vi "ScoutingMain.vi"() -> ()   [LabVIEW 2017]
uses:
  <vilib>/Utility/NIReport.llb/Append Report Text (str wrap).vi
  <vilib>/Utility/NIReport.llb/Append Image to Report (path wrap).vi
  <vilib>/Utility/config.llb/Read Key (Boolean).vi
  <vilib>/Utility/NIReport.llb/NI_report.lvclass
  <vilib>/Utility/config.llb/NI_LVConfig.lvlib
  <vilib>/zip/NI_Unzip.lvlib
  <vilib>/Utility/NIReport.llb/NI_ReportGenerationCore.lvlib
panel:
  in  "Export PDF":bool
  in  "Export":bool
  in  "Import":bool
  in  "Query":bool
  in  "Edit":bool
  in  "LookUp":bool
  in  "QR":bool
  in  "Snapshot":bool
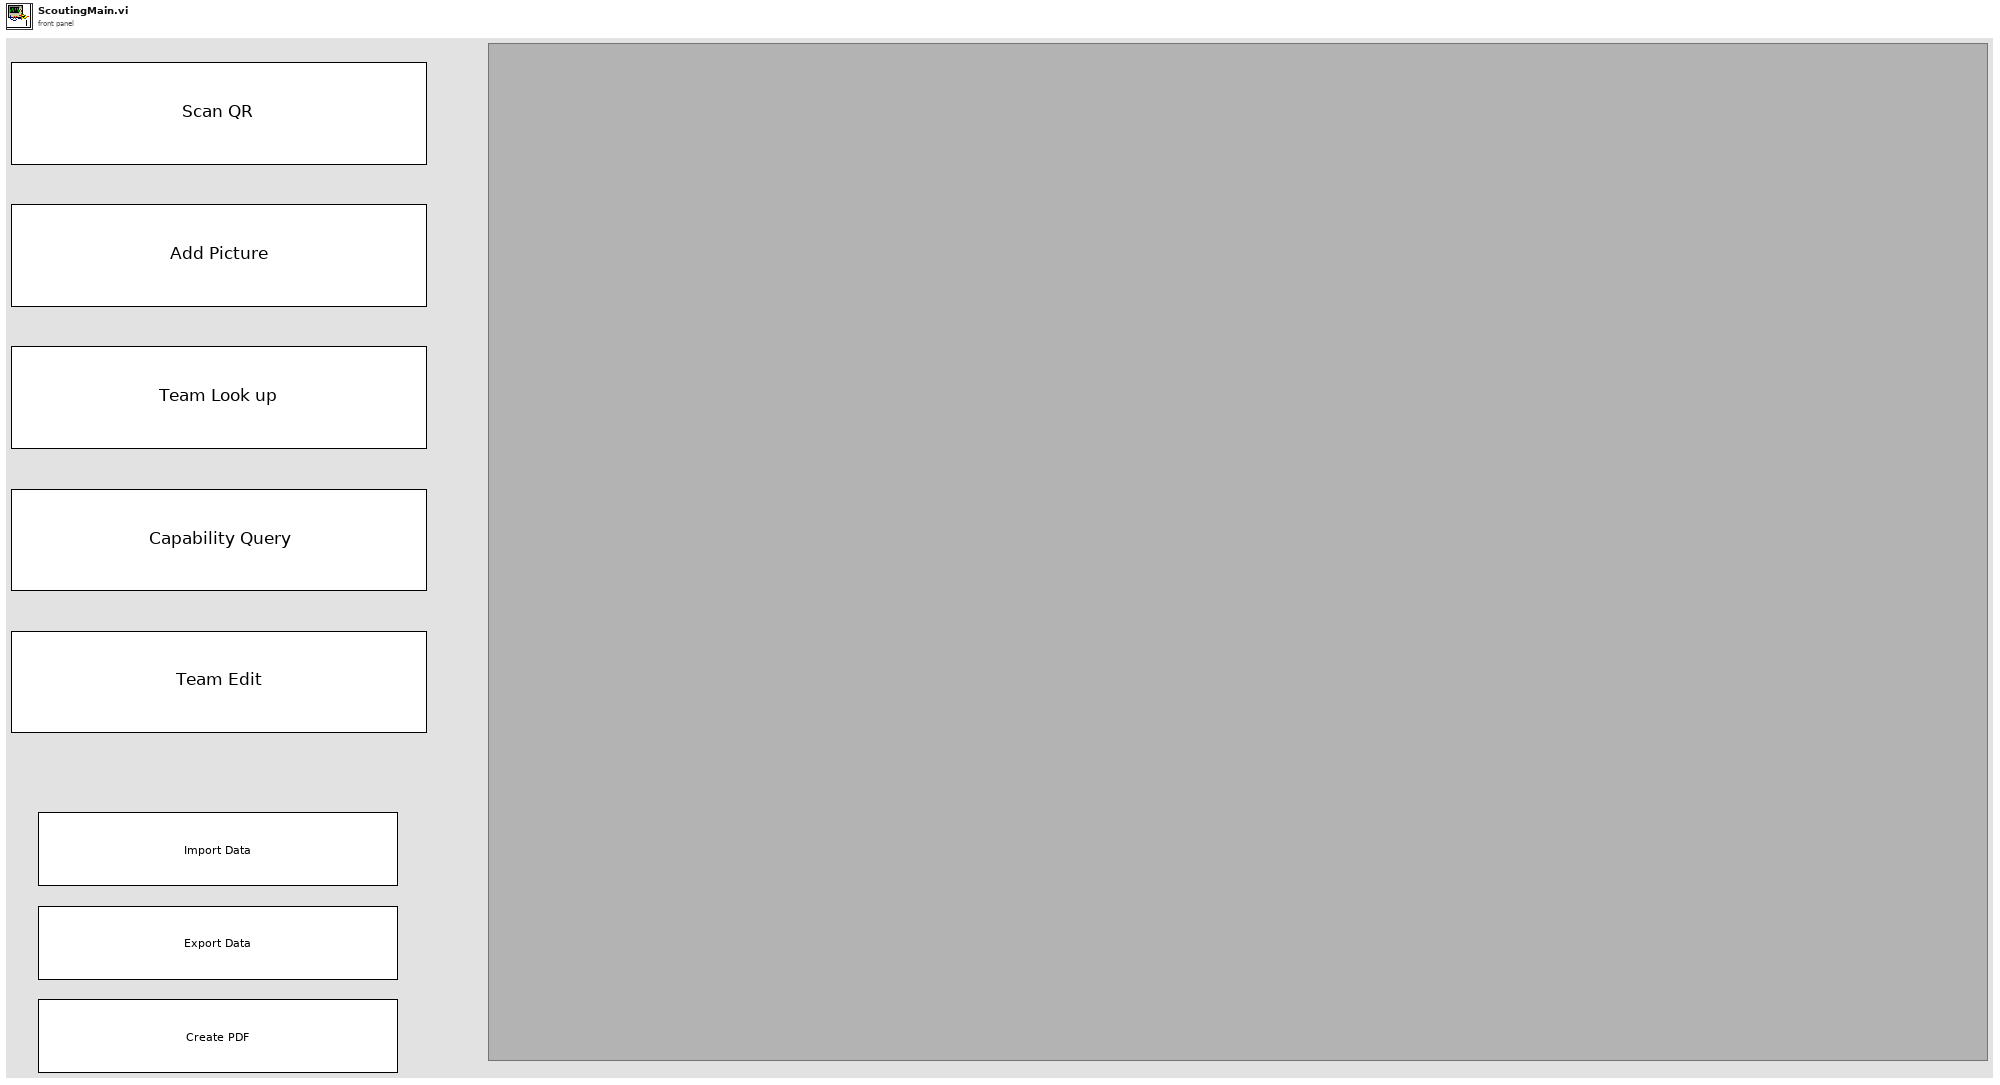
[diagram p1: front panel]
types:
  T1 = enum8{"Enabled", "Disabled", "Disabled and Grayed Out"}
  T2 = enum32{"invalid app kind", "Development System", "Run Time System", "Student Edition", "Embedded LabVIEW", "Evaluation", "Custom"}
  T3 = enum16{"Standard Report", "HTML", "Word", "Excel"}
  T4 = typedef "NI_LVConfig.lvlib/Config Data RefNum.ctl" = refnum<k1>
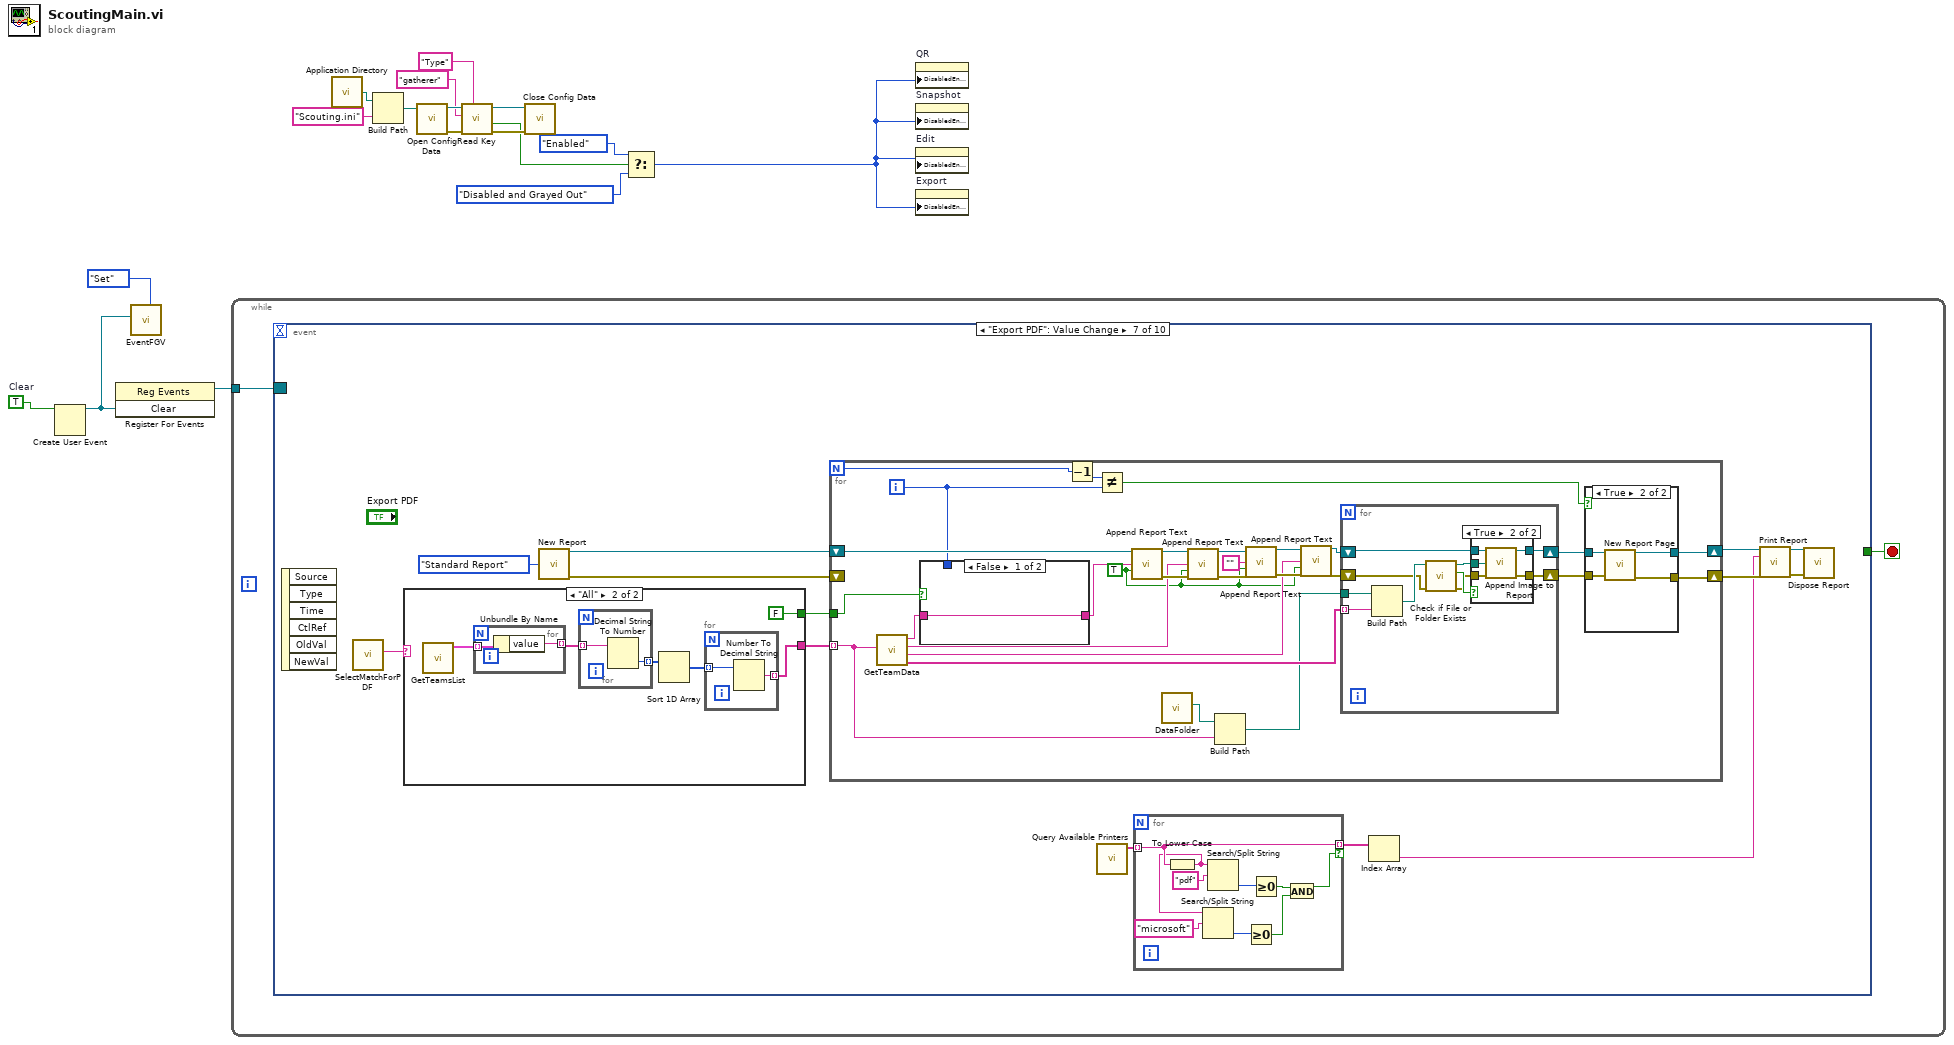
[diagram p0: block diagram]
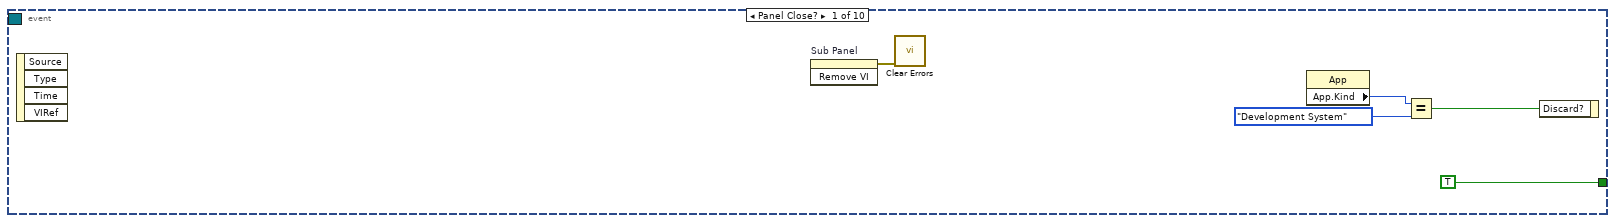
[diagram p2: hidden frame]
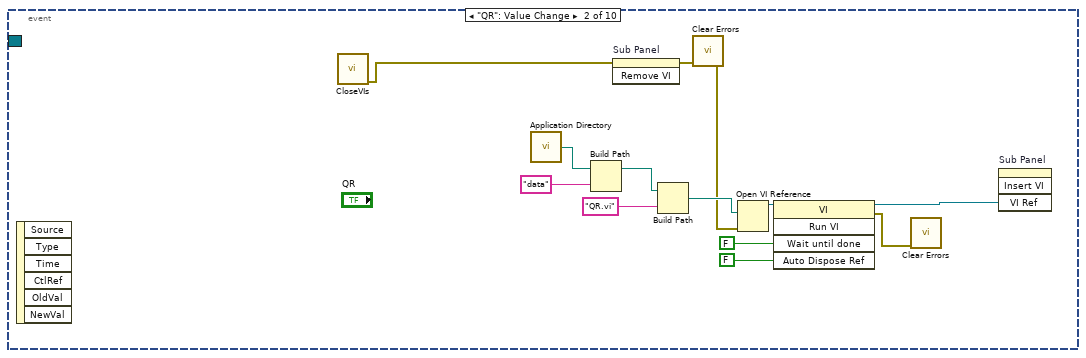
[diagram p3: hidden frame]
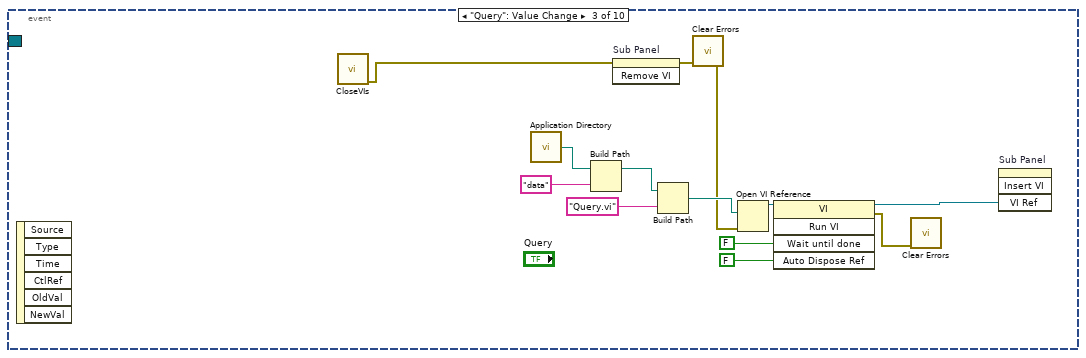
[diagram p4: hidden frame]
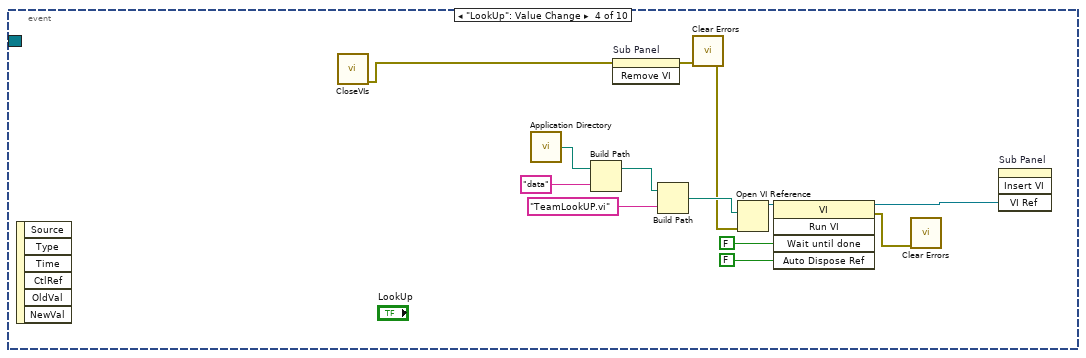
[diagram p5: hidden frame]
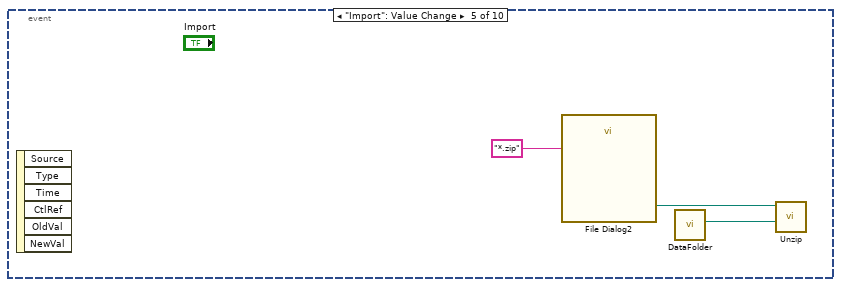
[diagram p6: hidden frame]
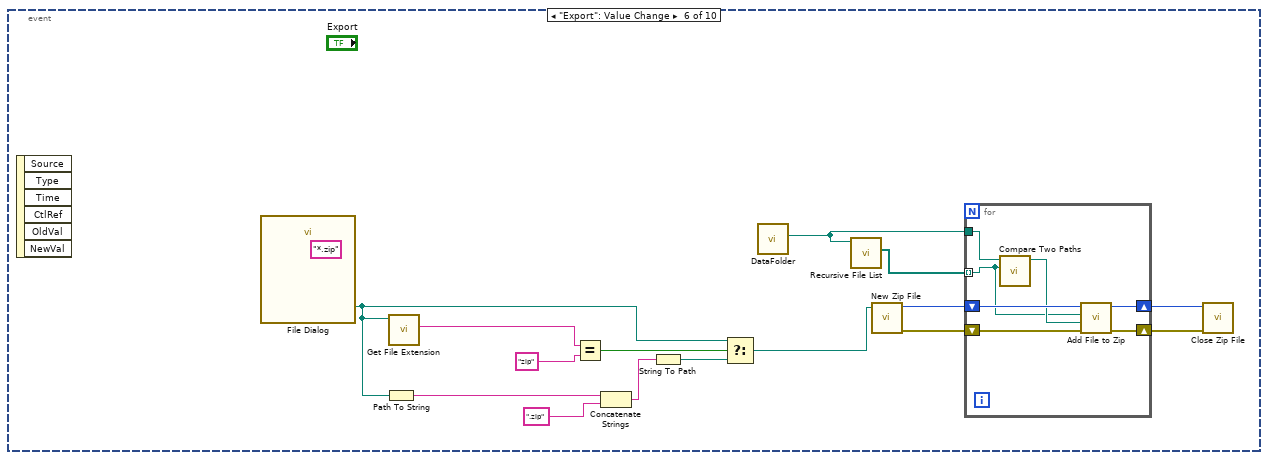
[diagram p7: hidden frame]
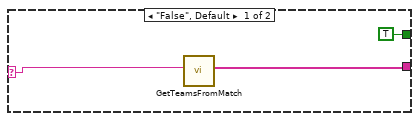
[diagram p8: hidden frame]
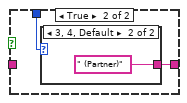
[diagram p9: hidden frame]
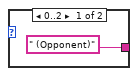
[diagram p10: hidden frame]
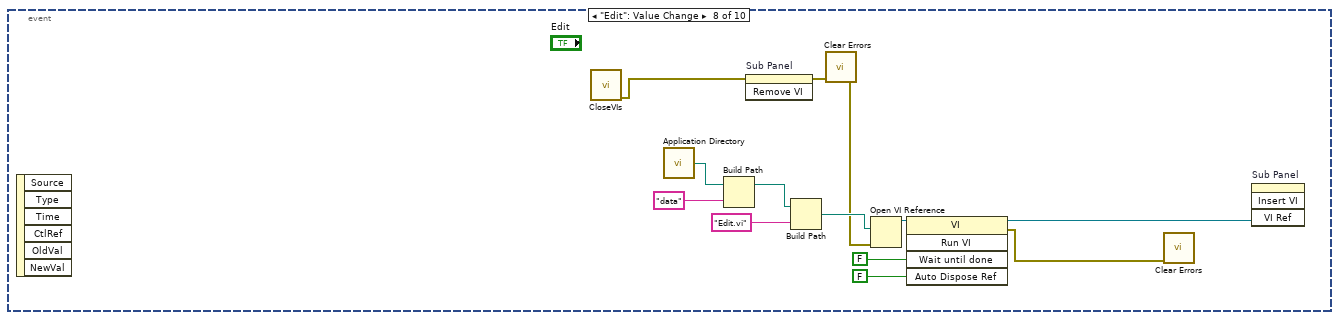
[diagram p13: hidden frame]
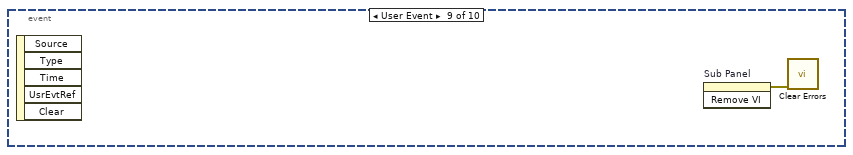
[diagram p14: hidden frame]
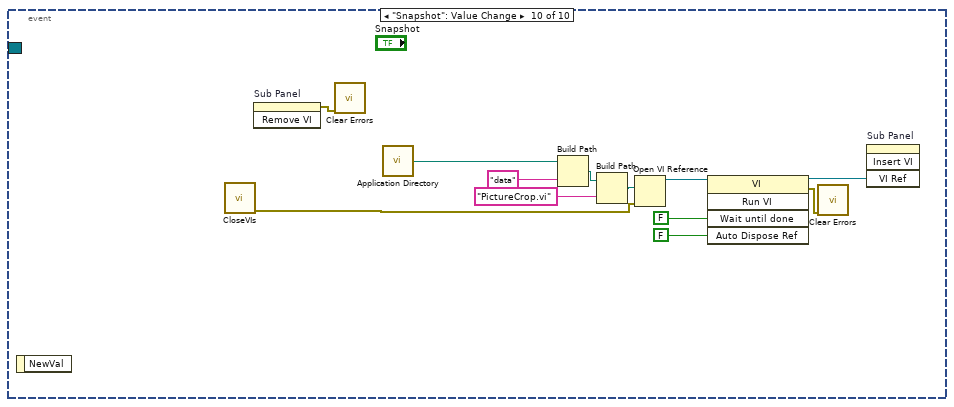
[diagram p15: hidden frame]
diagram:
  w17 = TRUE  # Clear
  n1 = Create User Event(user event datatype=w17) -> (user event=w15:refnum<user-event>)  [unwired: 1 in, 1 out]
  n2 = register-events(w15) -> (reference out=w16:refnum<event-registration>)  [unwired: 2 in, 1 out]
  n3 = call "EventFGV.vi"("Action"=enum16{"Set", "Get"}."Set", "user event in"=w15) -> ()  [unwired: 9 in, 1 out]
  n4 = while {
    tunnel: w16 -> [w18]
    stop <- w19 stop-if-true
    n5 = event shown="[6] \"Export PDF\": Value Change" {
      selector: w18 -> [_ _ _ _ _ _ _ _ _ _]
      dyn-events: _ -> [_ _ _ _ _ _ _ _ _ _]
      timeout: _ -> [_ _ _ _ _ _ _ _ _ _]
      tunnel: [TRUE _ _ _ _ _ _ _ _ _] -> w19
      event Panel Close? {
        n6 = event-data() -> ()  [unwired: 1 in, 4 out]
        n7 = invoke on="Sub Panel" class="SubPnl" method="Remove VI"() -> (error out=w20:errorcluster)  [unwired: 3 in, 2 out]
        n8 = call <vilib>:"Clear Errors.vi"("error in (no error)"=w20) -> ()  [unwired: 5 in, 2 out]
        n9 = property class="App"() -> ("App.Kind"=w23:T2)  [unwired: 2 in, 2 out]
        n10 = Equal?(x=w23, y=T2."Development System") -> (x = y?=w24:bool)
        n11 = event-data("Discard?"=w24) -> ()  [unwired: 1 in, 1 out]
      }
      event "QR": Value Change {
        n12 = event-data() -> ()  [unwired: 1 in, 6 out]
        n13 = call "CloseVIs.vi"() -> ("error out"=w25:errorcluster)  [unwired: 11 in]
        n14 = call <vilib>:"Application Directory.vi"() -> ("Application Directory"=w36:path)
        n15 = Build Path(base path=w36, name or relative path="data") -> (appended path=w30:path)
        n16 = invoke on="Sub Panel" class="SubPnl" method="Remove VI"(error in=w25) -> (error out=w27:errorcluster)  [unwired: 2 in, 2 out]
        n17 = Build Path(base path=w30, name or relative path="QR.vi") -> (appended path=w35:path)
        n18 = call <vilib>:"Clear Errors.vi"("error in (no error)"=w27) -> ("error out"=w26:errorcluster)  [unwired: 5 in, 1 out]
        n19 = Open VI Reference(vi path=w35, error in (no error)=w26) -> (vi reference=w37:refnum<vi>)  [unwired: 4 in, 1 out]
        n20 = invoke class="VI" method="Run VI"(reference=w37, "Wait until done"=FALSE ("Wait Until Done"), "Auto Dispose Ref"=FALSE ("Auto Dispose Reference")) -> (reference out=w33:refnum<vi>, error out=w28:errorcluster)  [unwired: 2 in, 3 out]
        n21 = call <vilib>:"Clear Errors.vi"("error in (no error)"=w28) -> ()  [unwired: 5 in, 2 out]
        n22 = invoke on="Sub Panel" class="SubPnl" method="Insert VI"("VI Ref"=w33) -> ()  [unwired: 3 in, 4 out]
      }
      event "Query": Value Change {
        n23 = event-data() -> ()  [unwired: 1 in, 6 out]
        n24 = call "CloseVIs.vi"() -> ("error out"=w38:errorcluster)  [unwired: 11 in]
        n25 = call <vilib>:"Application Directory.vi"() -> ("Application Directory"=w49:path)
        n26 = Build Path(base path=w49, name or relative path="data") -> (appended path=w43:path)
        n27 = invoke on="Sub Panel" class="SubPnl" method="Remove VI"(error in=w38) -> (error out=w40:errorcluster)  [unwired: 2 in, 2 out]
        n28 = Build Path(base path=w43, name or relative path="Query.vi") -> (appended path=w48:path)
        n29 = call <vilib>:"Clear Errors.vi"("error in (no error)"=w40) -> ("error out"=w39:errorcluster)  [unwired: 5 in, 1 out]
        n30 = Open VI Reference(vi path=w48, error in (no error)=w39) -> (vi reference=w50:refnum<vi>)  [unwired: 4 in, 1 out]
        n31 = invoke class="VI" method="Run VI"(reference=w50, "Wait until done"=FALSE ("Wait Until Done"), "Auto Dispose Ref"=FALSE ("Auto Dispose Reference")) -> (reference out=w46:refnum<vi>, error out=w41:errorcluster)  [unwired: 2 in, 3 out]
        n32 = call <vilib>:"Clear Errors.vi"("error in (no error)"=w41) -> ()  [unwired: 5 in, 2 out]
        n33 = invoke on="Sub Panel" class="SubPnl" method="Insert VI"("VI Ref"=w46) -> ()  [unwired: 3 in, 4 out]
      }
      event "LookUp": Value Change {
        n34 = event-data() -> ()  [unwired: 1 in, 6 out]
        n35 = call "CloseVIs.vi"() -> ("error out"=w51:errorcluster)  [unwired: 11 in]
        n36 = call <vilib>:"Application Directory.vi"() -> ("Application Directory"=w62:path)
        n37 = Build Path(base path=w62, name or relative path="data") -> (appended path=w56:path)
        n38 = invoke on="Sub Panel" class="SubPnl" method="Remove VI"(error in=w51) -> (error out=w53:errorcluster)  [unwired: 2 in, 2 out]
        n39 = Build Path(base path=w56, name or relative path="TeamLookUP.vi") -> (appended path=w61:path)
        n40 = call <vilib>:"Clear Errors.vi"("error in (no error)"=w53) -> ("error out"=w52:errorcluster)  [unwired: 5 in, 1 out]
        n41 = Open VI Reference(vi path=w61, error in (no error)=w52) -> (vi reference=w63:refnum<vi>)  [unwired: 4 in, 1 out]
        n42 = invoke class="VI" method="Run VI"(reference=w63, "Wait until done"=FALSE ("Wait Until Done"), "Auto Dispose Ref"=FALSE ("Auto Dispose Reference")) -> (reference out=w59:refnum<vi>, error out=w54:errorcluster)  [unwired: 2 in, 3 out]
        n43 = call <vilib>:"Clear Errors.vi"("error in (no error)"=w54) -> ()  [unwired: 5 in, 2 out]
        n44 = invoke on="Sub Panel" class="SubPnl" method="Insert VI"("VI Ref"=w59) -> ()  [unwired: 3 in, 4 out]
      }
      event "Import": Value Change {
        n45 = event-data() -> ()  [unwired: 1 in, 6 out]
        n46 = call "File Dialog2"("pattern (all files)"="*.zip") -> ("selected path"=w65:path)  [unwired: 11 in, 3 out]
        n47 = call "DataFolder.vi"() -> ("appended path"=w64:path)  [unwired: 11 in]
        n48 = call <vilib>:"Unzip.vi"("Target directory (same as Zip file if empty)"=w64, "Zip file"=w65) -> ()  [unwired: 7 in, 3 out]
      }
      event "Export": Value Change {
        n49 = event-data() -> ()  [unwired: 1 in, 6 out]
        n50 = call "File Dialog"("pattern (all files)"="*.zip") -> ("selected path"=w71:path)  [unwired: 11 in, 3 out]
        n51 = Path To String(path=w71) -> (string=w70:string)
        n52 = call <vilib>:"Get File Extension.vi"("file"=w71) -> ("lowercase file extension"=w74:string)  [unwired: 6 in, 4 out]
        n53 = Equal?(x=w74, y="zip") -> (x = y?=w73:bool)
        n54 = Concatenate Strings(w70, ".zip") -> (w68:string)
        n55 = String To Path(string=w68) -> (path=w67:path)
        n56 = Select(t=w71, s=w73, f=w67) -> (s? t:f=w72:path)
        n57 = call "DataFolder.vi"() -> ("appended path"=w78:path)  [unwired: 11 in]
        n58 = call <vilib>:"Recursive File List.vi"("Folder Path"=w78) -> ("All Files in Dir"=w77:path[])  [unwired: 6 in, 4 out]
        n59 = call <vilib>:"New Zip File.vi"("target"=w72) -> ("error out"=w80:errorcluster, "zip file out"=w81:i64)  [unwired: 4 in, 1 out]
        n60 = for {
          shift-right: [w89] -> w82
          shift-left: w81 -> [w88]
          shift-right: [w86] -> w79
          shift-left: w80 -> [w87]
          tunnel: w78 -> [w85]
          tunnel: w77 -> [w83] mode=indexing
          n61 = call <vilib>:"Compare Two Paths.vi"("Path 2"=w83, "Path 1"=w85) -> ("Relative Path from 1 to 2"=w84:path)  [unwired: 6 in, 3 out]
          n62 = call <vilib>:"Add File to Zip.vi"("error in (no error)"=w87, "destination path in zip"=w84, "source file path"=w83, "zip file in"=w88) -> ("error out"=w86:errorcluster, "zip file out"=w89:i64)  [unwired: 6 in]
        }
        n63 = call <vilib>:"Close Zip File.vi"("error in (no error)"=w79, "zip file in"=w82) -> ()  [unwired: 5 in, 1 out]
      }
      event "Export PDF": Value Change {
        n64 = event-data() -> ()  [unwired: 1 in, 6 out]
        n65 = call "SelectMatchForPDF.vi"() -> ("Select Teams 2"=w91:string)  [unwired: 11 in]
        n66 = case shown="\"All\"" w91 {
          selector: w91 -> [w105 _]
          tunnel: [w104 w108] -> w92
          tunnel: [TRUE FALSE] -> w90
          frame "False", Default {
            n67 = call "GetTeamsFromMatch.vi"("Match"=w105) -> ("Teams"=w104:string[])  [unwired: 10 in]
          }
          frame "All" {
            n68 = call "GetTeamsList.vi"() -> ("Array"=w107:cluster{string, "value":string}[])  [unwired: 11 in]
            n69 = for {
              tunnel: w107 -> [w113] mode=indexing
              tunnel: [w112] -> w111 mode=indexing
              n70 = Unbundle By Name(w113) -> ("value"=w112:string)
            }
            n71 = for {
              tunnel: w111 -> [w117] mode=indexing
              tunnel: [w116] -> w110 mode=indexing
              n72 = Decimal String To Number(string=w117) -> (number=w116:i32)  [unwired: 2 in, 1 out]
            }
            n73 = Sort 1D Array(array=w110) -> (sorted array=w109:i32[])
            n74 = for {
              tunnel: w109 -> [w115] mode=indexing
              tunnel: [w114] -> w108 mode=indexing
              n75 = Number To Decimal String(number=w115) -> (decimal integer string=w114:string)  [unwired: 1 in]
            }
          }
        }
        n76 = call <vilib>:"New Report.vi"("report type"=T3."Standard Report") -> ("report out"=w101:refnum<class "NI_report.lvclass">, "error out"=w100:errorcluster)  [unwired: 13 in]
        n77 = for {
          N -> [w151]
          tunnel: w92 -> [w131] mode=indexing
          shift-right: [w134] -> w97
          shift-left: w101 -> [w152]
          shift-right: [w133] -> w96
          shift-left: w100 -> [_]
          tunnel: w90 -> [w129]
          i -> [w127]
          w140 = TRUE ("append on new line? (F)")
          n78 = call "GetTeamData.vi"("Team #"=w131) -> ("Pictures"=w153:string[], "Data"=w141:string, "Location"=w147:string, "Name"=w130:string)  [unwired: 7 in]
          n79 = case shown="False" w129 {
            tunnel: w130 -> [w155 _]
            tunnel: [w155 w157] -> w128
            tunnel: w127 -> [_ w156]
            frame False {
            }
            frame True {
              n80 = case shown="3, 4, Default" w156 {
                tunnel: [" (Opponent)" " (Partner)"] -> w157
                frame 0..2 {
                }
                frame 3, 4, Default {
                }
              }
            }
          }
          n81 = Decrement(x=w151) -> (x-1=w150:i32)
          n82 = Not Equal?(x=w150, y=w127) -> (x != y?=w132:bool)
          n83 = call-poly <vilib>:"Append Report Text.vi"("report in"=w152, "text"=w128, "append on new line? (F)"=w140) -> ("report out"=w149:refnum<class "NI_report.lvclass">, "error out"=w148:errorcluster)  [unwired: 9 in, 2 out]
          n84 = call "DataFolder.vi"() -> ("appended path"=w154:path)  [unwired: 11 in]
          n85 = call-poly <vilib>:"Append Report Text.vi"("report in"=w149, "text"=w147, "append on new line? (F)"=w140, "error in (no error)"=w148) -> ("report out"=w146:refnum<class "NI_report.lvclass">, "error out"=w145:errorcluster)  [unwired: 8 in, 2 out]
          n86 = Build Path(base path=w154, name or relative path=w131) -> (appended path=w137:path)
          n87 = call-poly <vilib>:"Append Report Text.vi"("report in"=w146, "text"="", "append on new line? (F)"=w140, "error in (no error)"=w145) -> ("report out"=w143:refnum<class "NI_report.lvclass">, "error out"=w142:errorcluster)  [unwired: 8 in, 2 out]
          n88 = call-poly <vilib>:"Append Report Text.vi"("report in"=w143, "text"=w141, "append on new line? (F)"=w140, "error in (no error)"=w142) -> ("report out"=w138:refnum<class "NI_report.lvclass">, "error out"=w139:errorcluster)  [unwired: 8 in, 2 out]
          n89 = for {
            tunnel: w153 -> [w172] mode=indexing
            tunnel: w137 -> [w174]
            shift-right: [w171] -> w136
            shift-left: w138 -> [w175]
            shift-right: [w170] -> w135
            shift-left: w139 -> [w166]
            n90 = Build Path(base path=w174, name or relative path=w172) -> (appended path=w173:path)
            n91 = call <vilib>:"Check if File or Folder Exists.vi"("error in (no error)"=w166, "path"=w173) -> ("error out"=w167:errorcluster, "file or folder exists?"=w168:bool, "dup path"=w169:path)  [unwired: 7 in]
            n92 = case shown="True" w168 {
              tunnel: w167 -> [w176 w182]
              tunnel: w175 -> [w177 w181]
              tunnel: w169 -> [_ w180]
              tunnel: [w177 w179] -> w171
              tunnel: [w176 w178] -> w170
              frame False {
              }
              frame True {
                n93 = call-poly <vilib>:"Append Image to Report.vi"("report in"=w181, "path or URL of image"=w180, "error in (no error)"=w182) -> ("report out"=w179:refnum<class "NI_report.lvclass">, "error out"=w178:errorcluster)  [unwired: 9 in, 2 out]
              }
            }
          }
          n94 = case shown="True" w132 {
            tunnel: w136 -> [w161 w165]
            tunnel: w135 -> [w160 w164]
            tunnel: [w161 w163] -> w134
            tunnel: [w160 w162] -> w133
            frame False {
            }
            frame True {
              n95 = call-dynamic "New Report Page.vi"("report in"=w165, "error in (no error)"=w164) -> ("report out"=w163:refnum<class "NI_report.lvclass">, "error out"=w162:errorcluster)  [unwired: 12 in]
            }
          }
        }
        n96 = call <vilib>:"Query Available Printers.vi"() -> ("system configured printers"=w98:string[])  [unwired: 9 in, 2 out]
        n97 = for {
          tunnel: w98 -> [w125] mode=indexing
          tunnel: [w125] -> w99 mode=indexing if=w123
          n98 = To Lower Case(string=w125) -> (all lower case string=w120:string)
          n99 = Search/Split String(string=w120, search string/char (-)="microsoft") -> (offset of match=w122:i32)  [unwired: 1 in, 2 out]
          n100 = Search/Split String(string=w120, search string/char (-)="pdf") -> (offset of match=w126:i32)  [unwired: 1 in, 2 out]
          n101 = Greater Or Equal To 0?(x=w122) -> (x >= 0?=w118:bool)
          n102 = Greater Or Equal To 0?(x=w126) -> (x >= 0?=w124:bool)
          n103 = And(x=w124, y=w118) -> (x .and. y?=w123:bool)
        }
        n104 = Index Array(array=w99) -> (element=w95:string)  [unwired: 1 in]
        n105 = call-dynamic "Print Report.vi"("report in"=w97, "printer name (default)"=w95, "error in (no error)"=w96) -> ("report out"=w94:refnum<class "NI_report.lvclass">, "error out"=w93:errorcluster)  [unwired: 11 in]
        n106 = call-dynamic "Dispose Report.vi"("report in"=w94, "error in (no error)"=w93) -> ()  [unwired: 13 in, 1 out]
      }
      event "Edit": Value Change {
        n107 = event-data() -> ()  [unwired: 1 in, 6 out]
        n108 = call "CloseVIs.vi"() -> ("error out"=w189:errorcluster)  [unwired: 11 in]
        n109 = call <vilib>:"Application Directory.vi"() -> ("Application Directory"=w194:path)
        n110 = Build Path(base path=w194, name or relative path="data") -> (appended path=w192:path)
        n111 = invoke on="Sub Panel" class="SubPnl" method="Remove VI"(error in=w189) -> (error out=w191:errorcluster)  [unwired: 2 in, 2 out]
        n112 = Build Path(base path=w192, name or relative path="Edit.vi") -> (appended path=w193:path)
        n113 = call <vilib>:"Clear Errors.vi"("error in (no error)"=w191) -> ("error out"=w190:errorcluster)  [unwired: 5 in, 1 out]
        n114 = Open VI Reference(vi path=w193, error in (no error)=w190) -> (vi reference=w195:refnum<vi>)  [unwired: 4 in, 1 out]
        n115 = invoke class="VI" method="Run VI"(reference=w195, "Wait until done"=FALSE ("Wait Until Done"), "Auto Dispose Ref"=FALSE ("Auto Dispose Reference")) -> (reference out=w183:refnum<vi>, error out=w184:errorcluster)  [unwired: 2 in, 3 out]
        n116 = call <vilib>:"Clear Errors.vi"("error in (no error)"=w184) -> ()  [unwired: 5 in, 2 out]
        n117 = invoke on="Sub Panel" class="SubPnl" method="Insert VI"("VI Ref"=w183) -> ()  [unwired: 3 in, 4 out]
      }
      event User Event {
        n118 = event-data() -> ()  [unwired: 1 in, 5 out]
        n119 = invoke on="Sub Panel" class="SubPnl" method="Remove VI"() -> (error out=w196:errorcluster)  [unwired: 3 in, 2 out]
        n120 = call <vilib>:"Clear Errors.vi"("error in (no error)"=w196) -> ()  [unwired: 5 in, 2 out]
      }
      event "Snapshot": Value Change {
        n121 = event-data() -> ()  [unwired: 1 in, 1 out]
        n122 = call "CloseVIs.vi"() -> ("error out"=w197:errorcluster)  [unwired: 11 in]
        n123 = invoke on="Sub Panel" class="SubPnl" method="Remove VI"() -> (error out=w198:errorcluster)  [unwired: 3 in, 2 out]
        n124 = call <vilib>:"Clear Errors.vi"("error in (no error)"=w198) -> ()  [unwired: 5 in, 2 out]
        n125 = call <vilib>:"Application Directory.vi"() -> ("Application Directory"=w201:path)
        n126 = Build Path(base path=w201, name or relative path="data") -> (appended path=w200:path)
        n127 = Build Path(base path=w200, name or relative path="PictureCrop.vi") -> (appended path=w207:path)
        n128 = Open VI Reference(vi path=w207, error in (no error)=w197) -> (vi reference=w208:refnum<vi>)  [unwired: 4 in, 1 out]
        n129 = invoke class="VI" method="Run VI"(reference=w208, "Wait until done"=FALSE ("Wait Until Done"), "Auto Dispose Ref"=FALSE ("Auto Dispose Reference")) -> (reference out=w205:refnum<vi>, error out=w199:errorcluster)  [unwired: 2 in, 3 out]
        n130 = call <vilib>:"Clear Errors.vi"("error in (no error)"=w199) -> ()  [unwired: 5 in, 2 out]
        n131 = invoke on="Sub Panel" class="SubPnl" method="Insert VI"("VI Ref"=w205) -> ()  [unwired: 3 in, 4 out]
      }
    }
  }
  n132 = call <vilib>:"Application Directory.vi"() -> ("Application Directory"=w13:path)
  n133 = Build Path(base path=w13, name or relative path="Scouting.ini") -> (appended path=w11:path)
  n134 = call <vilib>:"Open Config Data.vi"("configuration file path"=w11) -> ("error out"=w10:errorcluster, "refnum"=w9:T4)  [unwired: 8 in, 1 out]
  n135 = call-poly <vilib>:"Read Key.vi"("section"="Type", "error in (no error)"=w10, "key"="gatherer", "refnum"=w9) -> ("error out"=w6:errorcluster, "value"=w4:bool, "refnum out"=w5:T4)  [unwired: 4 in, 1 out]
  n136 = call <vilib>:"Close Config Data.vi"("error in (no error)"=w6, "refnum"=w5) -> ()  [unwired: 8 in, 2 out]
  n137 = Select(t=T1."Enabled" ("Disabled"), s=w4, f=T1."Disabled and Grayed Out") -> (s? t:f=w1:T1)
  n138 = property on="QR" class="Bool"("DisabledEnum"=w1) -> ()  [unwired: 2 in, 2 out]
  n139 = property on="Snapshot" class="Bool"("DisabledEnum"=w1) -> ()  [unwired: 2 in, 2 out]
  n140 = property on="Edit" class="Bool"("DisabledEnum"=w1) -> ()  [unwired: 2 in, 2 out]
  n141 = property on="Export" class="Bool"("DisabledEnum"=w1) -> ()  [unwired: 2 in, 2 out]
